vi "Create TableColumns.vi"(8 "error in":errorcluster, 11 "Header Names":string[](array[string])) -> (0 "error out":errorcluster, 3 "TableColumns":refnum<k24>)   [LabVIEW 2019, in "Open Xml.lvlib"]
uses:
  Open Xml.lvlib
  D:/git/Open-Xml-LabVIEW/Source/DocumentFormat.OpenXml.dll
  DocumentFormat.OpenXml.dll
  D:/git/Open-Xml-LabVIEW/Source/DocumentFormat.OpenXml.Framework.dll
  DocumentFormat.OpenXml.Framework.dll
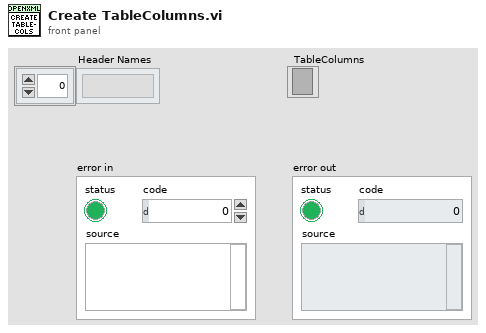
[diagram p1: front panel]
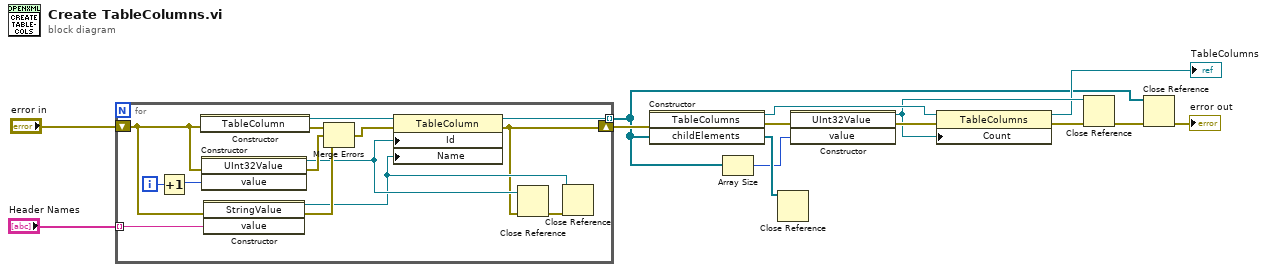
[diagram p0: block diagram]
diagram:
  n1 = for {
    tunnel: "Header Names" -> [w16] mode=indexing
    tunnel: [w27] -> w2 mode=indexing
    shift-right: [w15] -> w6
    shift-left: "error in" -> [w17]
    i -> [w25]
    n2 = Increment(x=w25) -> (x+1=w24:i32)
    n3 = constructor class="TableColumn"(error in=w17) -> (reference out=w28:refnum<k24>, error out=w26:errorcluster)  [unwired: 2 in, 1 out]
    n4 = constructor class="UInt32Value"(error in=w17, "value"=w24) -> (reference out=w19:refnum<k24>, error out=w22:errorcluster)  [unwired: 2 in, 2 out]
    n5 = constructor class="StringValue"(error in=w17, "value"=w16) -> (reference out=w18:refnum<k24>, error out=w21:errorcluster)  [unwired: 2 in, 2 out]
    n6 = Merge Errors(w26, w22, w21) -> (w23:errorcluster)
    n7 = property class="TableColumn"(reference=w28, error in=w23, "Id"=w19, "Name"=w18) -> (reference out=w27:refnum<k24>, error out=w15:errorcluster)
    n8 = Close Reference(reference=w19, error in (no error)=w15) -> (error out=w20:errorcluster)
    n9 = Close Reference(reference=w18, error in (no error)=w20) -> ()  [unwired: 1 out]
  }
  n10 = constructor class="TableColumns"(error in=w6, "childElements"=w2) -> (reference out=w8:refnum<k24>, error out=w9:errorcluster, "childElements"=w12:refnum<k24>[])  [unwired: 2 in, 1 out]
  n11 = Array Size(array=w2) -> (size(s)=w11:i32)
  n12 = Close Reference(reference=w12) -> ()  [unwired: 1 in, 1 out]
  n13 = constructor class="UInt32Value"(error in=w9, "value"=w11) -> (reference out=w4:refnum<k24>, error out=w10:errorcluster)  [unwired: 2 in, 2 out]
  n14 = property class="TableColumns"(reference=w8, error in=w10, "Count"=w4) -> (reference out=→"TableColumns":refnum<k24>, error out=w7:errorcluster)
  n15 = Close Reference(reference=w4, error in (no error)=w7) -> (error out=w5:errorcluster)
  n16 = Close Reference(reference=w2, error in (no error)=w5) -> (error out=→"error out":errorcluster)
